vi "get min max.vi"(8 "error in (no error)":errorcluster, 11 "LineCCD in":refnum<class "LineCCD.lvclass">) -> (0 "error out":errorcluster, 3 "LineCCD out":refnum<class "LineCCD.lvclass">)   [LabVIEW 2012, in "LineCCD.lvclass"]
uses:
  LineCCD.lvclass
  LineCCD.lvclass/LineCCD.ctl
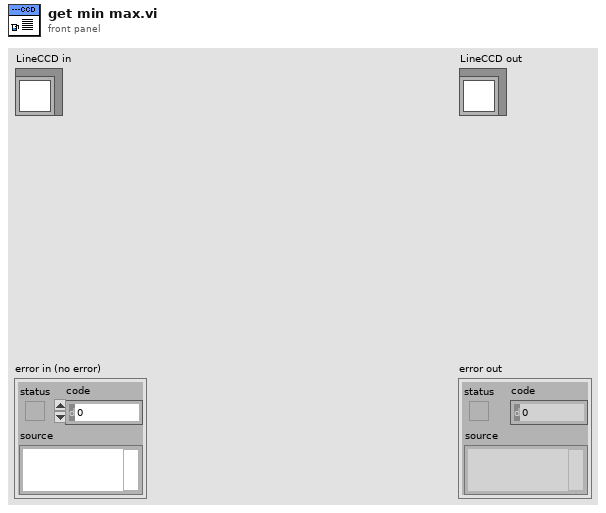
[diagram p1: front panel]
types:
  T1 = cluster{"[0]":i32, "[1]":i32, "[2]":i32, "[3]":i32, "[4]":i32, "[5]":i32, "[6]":i32, "[7]":i32}
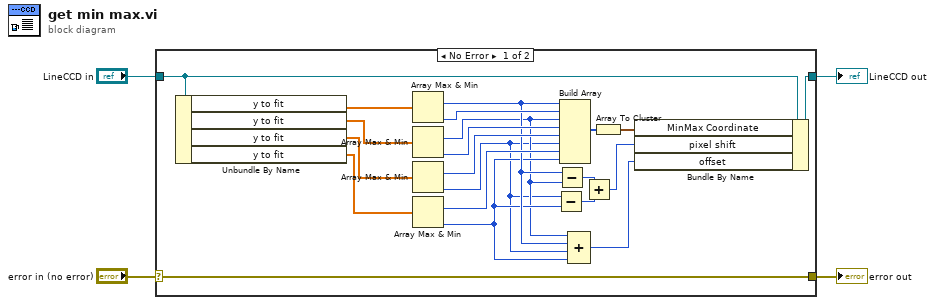
[diagram p0: block diagram]
diagram:
  n1 = case shown="No Error" "error in (no error)" {
    selector: "error in (no error)" -> [w25 w27]
    tunnel: [w25 w27] -> w3
    tunnel: [w20 w26] -> w1
    tunnel: "LineCCD in" -> [w21 w26]
    frame No Error {
      n2 = Unbundle By Name(w21) -> ("y to fit"=w23:dbl[], "y to fit"=w24:dbl[], "y to fit"=w14:dbl[], "y to fit"=w13:dbl[])
      n3 = Array Max & Min(array=w23) -> (max index (indices)=w10:i32, min index (indices)=w19:i32)  [unwired: 2 out]
      n4 = Array Max & Min(array=w24) -> (max index (indices)=w6:i32, min index (indices)=w18:i32)  [unwired: 2 out]
      n5 = Array Max & Min(array=w14) -> (max index (indices)=w17:i32, min index (indices)=w5:i32)  [unwired: 2 out]
      n6 = Array Max & Min(array=w13) -> (max index (indices)=w16:i32, min index (indices)=w9:i32)  [unwired: 2 out]
      n7 = Subtract(x=w5, y=w9) -> (x-y=w11:i32)
      n8 = Subtract(x=w10, y=w6) -> (x-y=w12:i32)
      n9 = Build Array(w10, w19, w6, w18, w17, w5, w16, w9) -> (w22:i32[])
      n10 = Compound Arithmetic op=ADD(w6, w10, w5, w9) -> (w7:i32)
      n11 = Add(x=w12, y=w11) -> (x+y=w8:i32)
      n12 = Array To Cluster(array=w22) -> (cluster=w15:T1)
      n13 = Bundle By Name(cluster=w21, "MinMax Coordinate"=w15, "pixel shift"=w8, "offset"=w7) -> (w20:refnum<class "LineCCD.lvclass">)
    }
    frame Error {
    }
  }
  "error out" <- w3
  "LineCCD out" <- w1
